vi "LWXPS_SingleAxisThetaPositionRawGet.vi"(0 "XPS Reference IN":refnum<k24>, 7 "Group Name":string, 11 "LabVIEW error IN":errorcluster) -> (3 "XPS Reference OUT":refnum<k24>, 4 "Returned error code":i32, 6 "Raw encoder position 1":dbl, 8 "Raw encoder position 2":dbl, 10 "Raw encoder position 3":dbl, 14 "LabVIEW error OUT":errorcluster, 15 "XPS Error String":string)   [LabVIEW 2014]
uses:
  D:/XPSQ8_LabView_Library/Development/Source/Dll/Newport.XPS.CommandInterface.dll
  Dll/Newport.XPS.CommandInterface.dll
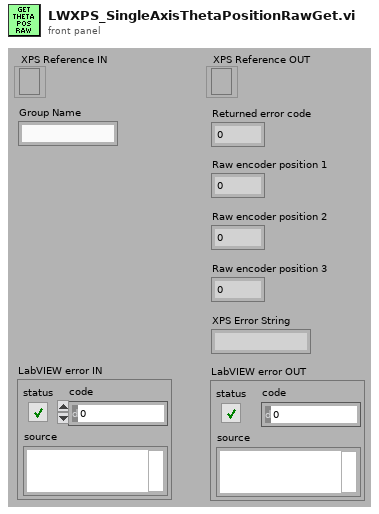
[diagram p1: front panel]
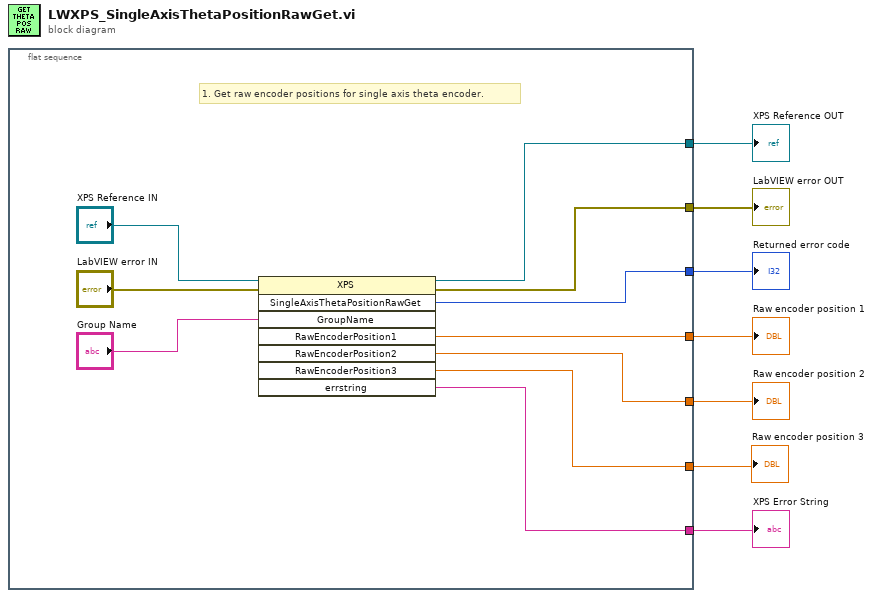
[diagram p0: block diagram]
diagram:
  n1 = flat-sequence {
    tunnel: [w15] -> w7
    tunnel: [w13] -> w6
    tunnel: [w16] -> w5
    tunnel: [w11] -> w3
    tunnel: [w12] -> w4
    tunnel: [w10] -> w1
    tunnel: [w9] -> w2
    frame #0 {
      # "1. Get raw encoder positions for single axis theta encoder."
      n2 = invoke class="XPS" method="SingleAxisThetaPositionRawGet"(reference="XPS Reference IN", error in="LabVIEW error IN", "GroupName"="Group Name") -> (reference out=w15:refnum<k24>, error out=w13:errorcluster, "SingleAxisThetaPositionRawGet"=w16:i32, "RawEncoderPosition1"=w11:dbl, "RawEncoderPosition2"=w12:dbl, "RawEncoderPosition3"=w10:dbl, "errstring"=w9:string)  [unwired: 5 in, 1 out]
    }
  }
  "XPS Error String" <- w2
  "XPS Reference OUT" <- w7
  "LabVIEW error OUT" <- w6
  "Returned error code" <- w5
  "Raw encoder position 2" <- w4
  "Raw encoder position 1" <- w3
  "Raw encoder position 3" <- w1
